vi "avoidCollideBall.vi"(0 "KickToSkill in":refnum<class "KickToSkill.lvclass">, 1 "AttackerAngle\nToTurnInDegrees":dbl, 3 "DistanceToGoAroundBall":dbl=200.0, 5 "Robot":refnum<class "Robot.lvclass">, 9 "Ball":refnum<class "Ball.lvclass">, 11 "error in (no error)":errorcluster, 12 "firstCallForState":bool, 13 "Target":dbl[](array[numeric]), 14 "DistanceToConsiderRobotArrive":dbl) -> (4 "KickToSkill out":refnum<class "KickToSkill.lvclass">, 6 "Robot out":refnum<class "Robot.lvclass">, 10 "robotKickState":T1=enum."avoidCollideBall", 15 "error out":errorcluster)   [LabVIEW 2023, in "KickToSkill.lvclass"]
uses:
  KickToSkill.lvclass
  Ball_class/Ball.lvclass
  C:/Users/lucio/Desktop/roboime/SSL_AI/Object_class/Object.lvclass
  Robot_class/Robot.lvclass
  Robot_class/robotKickToStates.ctl
  Object_class/Object.lvclass/Object.ctl
  Robot_class/Robot.lvclass/Robot.ctl
  <vilib>/Analysis/baseanly.llb/Unit Vector (DBL).vi
  <vilib>/Analysis/coordinate.llb/2D Cartesian Coordinate Rotation (Scalar).vi
  Object_class/Read position(x,y).vi
  Robot_class/Write dest_x.vi
  Robot_class/Write dest_y.vi
  Robot_class/Write dest_orientation.vi
  Utilities_class/Utilities.lvclass
  <vilib>/Analysis/NI_AALBase.lvlib
  <vilib>/Analysis/NI_AALPro.lvlib
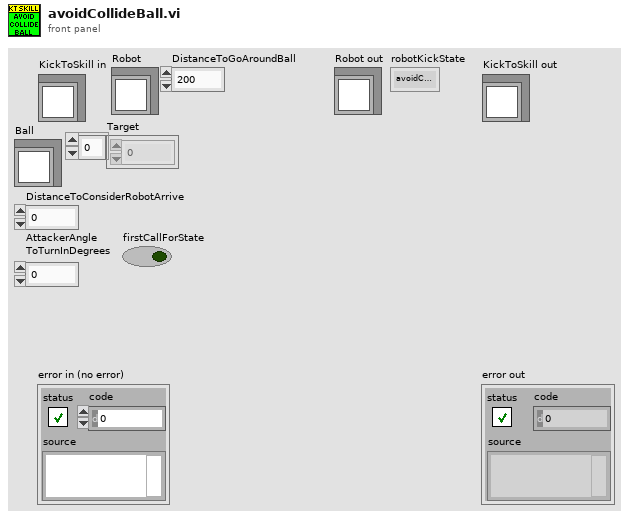
[diagram p1: front panel]
types:
  T1 = typedef "robotKickToStates.ctl" = enum16{"shootFromDirect", "avoidCollideBall", "goToBackBall", "none", "walk", "turn", "turnAntiClockWise", "turnClockwise", "oldKickToShoot", "oldKickToGoToBackBall", "shoot"}
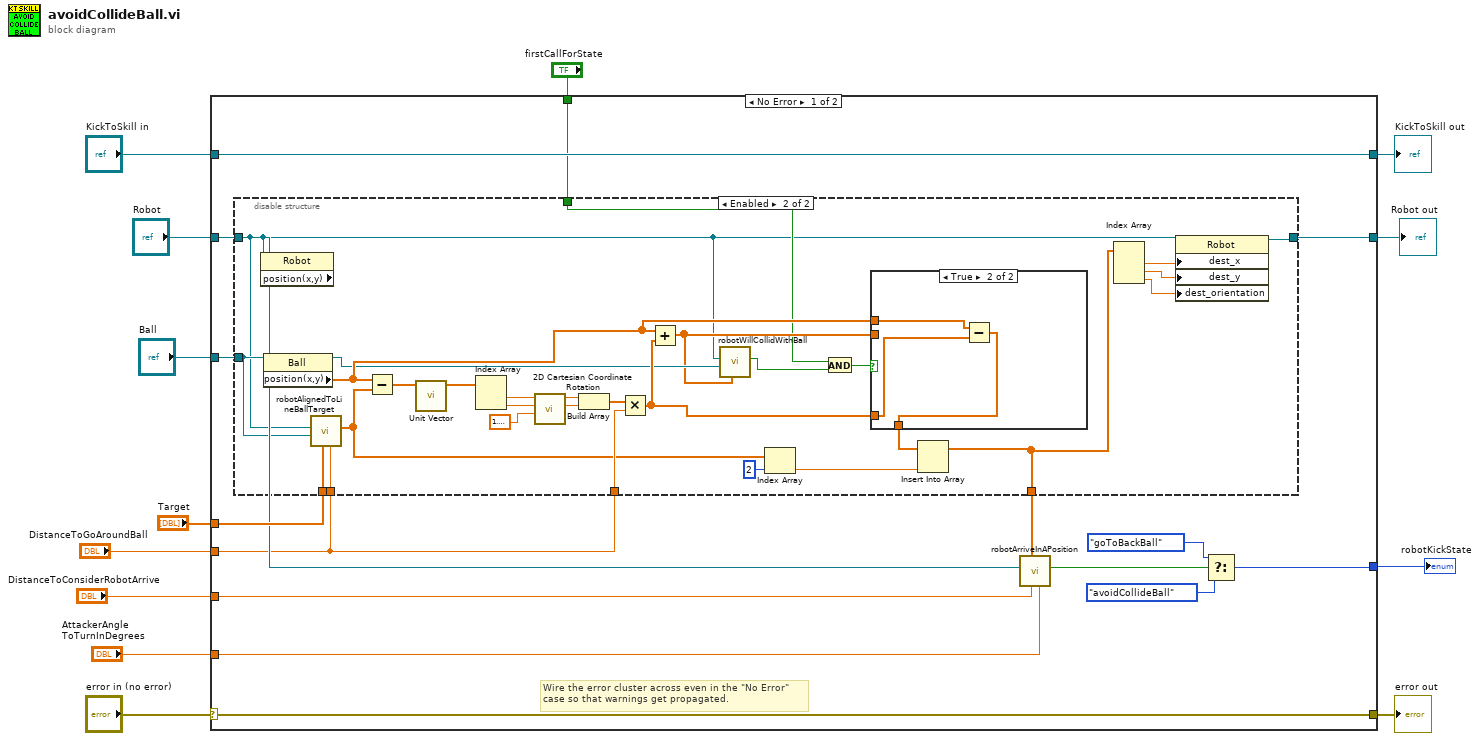
[diagram p0: block diagram]
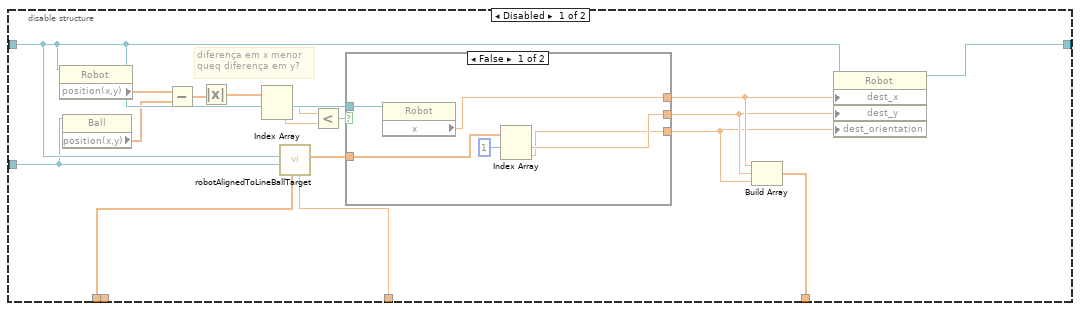
[diagram p2: hidden frame]
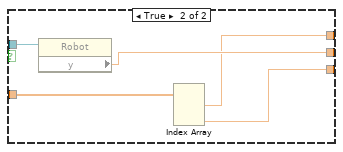
[diagram p3: hidden frame]
diagram:
  n1 = case shown="No Error" "error in (no error)" {
    selector: "error in (no error)" -> [w27 w91]
    tunnel: [w27 w91] -> w12
    tunnel: [w28 w90] -> w10
    tunnel: "KickToSkill in" -> [w28 w90]
    tunnel: "Ball" -> [w21 _]
    tunnel: "Target" -> [w26 _]
    tunnel: "Robot" -> [w22 _]
    tunnel: [w25 _] -> w6
    tunnel: [w14 _] -> w5
    tunnel: "DistanceToConsiderRobotArrive" -> [w19 _]
    tunnel: "AttackerAngle\nToTurnInDegrees" -> [w18 _]
    tunnel: "DistanceToGoAroundBall" -> [w17 _]
    tunnel: "firstCallForState" -> [w16 _]
    frame No Error {
      # "Wire the error cluster across even in the \"No Error\"\ncase so that warnings get propagated."
      n2 = disable-structure shown="Enabled" {
        disable-tunnel: w26 -> [w45 w63]
        disable-tunnel: [w44 w74] -> w25
        disable-tunnel: w22 -> [w42 w58]
        disable-tunnel: w21 -> [w41 w68]
        disable-tunnel: [w30 w73] -> w20
        disable-tunnel: w17 -> [w29 w77]
        disable-tunnel: w17 -> [_ w69]
        disable-tunnel: w16 -> [_ w59]
        frame Disabled {
          # "diferença em x menor\nqueq diferença em y?"
          n3 = property class="Robot"(reference=w42) -> ("position(x,y)"=w40:dbl[])  [unwired: 1 in, 2 out]
          n4 = property class="Ball"(reference=w41) -> ("position(x,y)"=w39:dbl[])  [unwired: 1 in, 2 out]
          n5 = Subtract(x=w40, y=w39) -> (x-y=w38:dbl[])
          n6 = Absolute Value(x=w38) -> (abs(x)=w37:dbl[])
          n7 = Index Array(array=w37) -> (element #1=w36:dbl, element #2=w35:dbl)  [unwired: 2 in]
          n8 = call "robotAlignedToLineBallTarget.vi"("DistanceToGoAroundBall"=w29, "Target"=w45, "Ball"=w41, "Robot in"=w42) -> ("dest(x, y, orientaion)"=w43:dbl[])  [unwired: 5 in, 2 out]
          n9 = Less?(x=w36, y=w35) -> (x < y?=w34:bool)
          n10 = case shown="False" w34 {
            tunnel: w43 -> [w50 w54]
            tunnel: [w49 w55] -> w32
            tunnel: [w48 w52] -> w31
            tunnel: w42 -> [w47 w56]
            tunnel: [w46 w53] -> w33
            frame False {
              n11 = property class="Robot"(reference=w47) -> ("x"=w46:dbl)  [unwired: 1 in, 2 out]
              n12 = Index Array(array=w50, index #1=1 ("index")) -> (element #1=w49:dbl, element #2=w48:dbl)  [unwired: 1 in]
            }
            frame True {
              n13 = property class="Robot"(reference=w56) -> ("y"=w55:dbl)  [unwired: 1 in, 2 out]
              n14 = Index Array(array=w54) -> (element #1=w53:dbl, element #3=w52:dbl)  [unwired: 3 in, 1 out]
            }
          }
          n15 = Build Array(w33, w32, w31) -> (w30:dbl[])
          n16 = property class="Robot"(reference=w42, "dest_x"=w33, "dest_y"=w32, "dest_orientation"=w31) -> (reference out=w44:refnum<class "Robot.lvclass">)  [unwired: 1 in, 1 out]
        }
        frame Enabled {
          n17 = property class="Robot" props=["position(x,y)"](reference=w58) -> ()  [unwired: 1 in, 3 out]
          n18 = property class="Ball"(reference=w68) -> (reference out=w64:refnum<class "Ball.lvclass">, "position(x,y)"=w65:dbl[])  [unwired: 1 in, 1 out]
          n19 = call "robotAlignedToLineBallTarget.vi"("DistanceToGoAroundBall"=w69, "Target"=w63, "Ball"=w68, "Robot in"=w58) -> ("dest(x, y, orientaion)"=w57:dbl[])  [unwired: 5 in, 2 out]
          n20 = Subtract(x=w65, y=w57) -> (x-y=w85:dbl[])
          n21 = call-poly <vilib>:"Unit Vector.vi"("Input Vector"=w85) -> ("Unit Vector"=w84:dbl[])  [unwired: 8 in, 2 out]
          n22 = Index Array(array=w84) -> (element #1=w83:dbl, element #2=w82:dbl)  [unwired: 2 in]
          n23 = call-poly <vilib>:"2D Cartesian Coordinate Rotation.vi"("theta"=1.5707963267948966, "y"=w82, "x"=w83) -> ("y out"=w79:dbl, "x out"=w80:dbl)  [unwired: 6 in, 1 out]
          n24 = Build Array(w80, w79) -> (w78:dbl[])
          n25 = Multiply(x=w78, y=w77) -> (x*y=w75:dbl[])
          n26 = Add(x=w65, y=w75) -> (x+y=w62:dbl[])
          n27 = call "robotWillCollidWithBall.vi"("target"=w62, "Ball"=w64, "Robot"=w58) -> ("robotCollideWithBall"=w60:bool)  [unwired: 6 in, 2 out]
          n28 = Index Array(array=w57, index=2) -> (element=w66:dbl)
          n29 = And(x=w59, y=w60) -> (x .and. y?=w61:bool)
          n30 = case shown="True" w61 {
            tunnel: [w86 w87] -> w76
            tunnel: w62 -> [w86 _]
            tunnel: w65 -> [_ w89]
            tunnel: w75 -> [_ w88]
            frame False {
            }
            frame True {
              n31 = Subtract(x=w89, y=w88) -> (x-y=w87:dbl[])
            }
          }
          n32 = Insert Into Array(array=w76, new element=w66) -> (w73:dbl[])  [unwired: 1 in]
          n33 = Index Array(array=w73) -> (element #1=w72:dbl, element #2=w71:dbl, element #3=w70:dbl)  [unwired: 3 in]
          n34 = property class="Robot"(reference=w58, "dest_x"=w72, "dest_y"=w71, "dest_orientation"=w70) -> (reference out=w74:refnum<class "Robot.lvclass">)  [unwired: 1 in, 1 out]
        }
      }
      n35 = call "robotArriveInAPosition.vi"("AttackerAngle\nToTurnInDegrees"=w18, "DistanceToConsiderRobotArrive"=w19, "Target(x, y, orientation)"=w20, "Robot"=w22) -> ("arrive?"=w24:bool)  [unwired: 5 in, 2 out]
      n36 = Select(t=robotKickToStates."goToBackBall" ("robotKickState"), s=w24, f=robotKickToStates."avoidCollideBall") -> (s? t:f=w14:T1)
    }
    frame Error {
    }
  }
  "error out" <- w12
  "KickToSkill out" <- w10
  "Robot out" <- w6
  "robotKickState" <- w5
